vi "RTS Read Point File.vi"(8 "Error In":errorcluster, 11 "Path":path) -> (0 "Error Out":errorcluster, 2 "Array 2":string[](array[string]), 3 "Point File":T1[](array[typedef]))   [LabVIEW 2018]
uses:
  Type Definitions/RTS Point File.ctl
  <vilib>/Utility/file.llb/Read Delimited Spreadsheet (string).vi
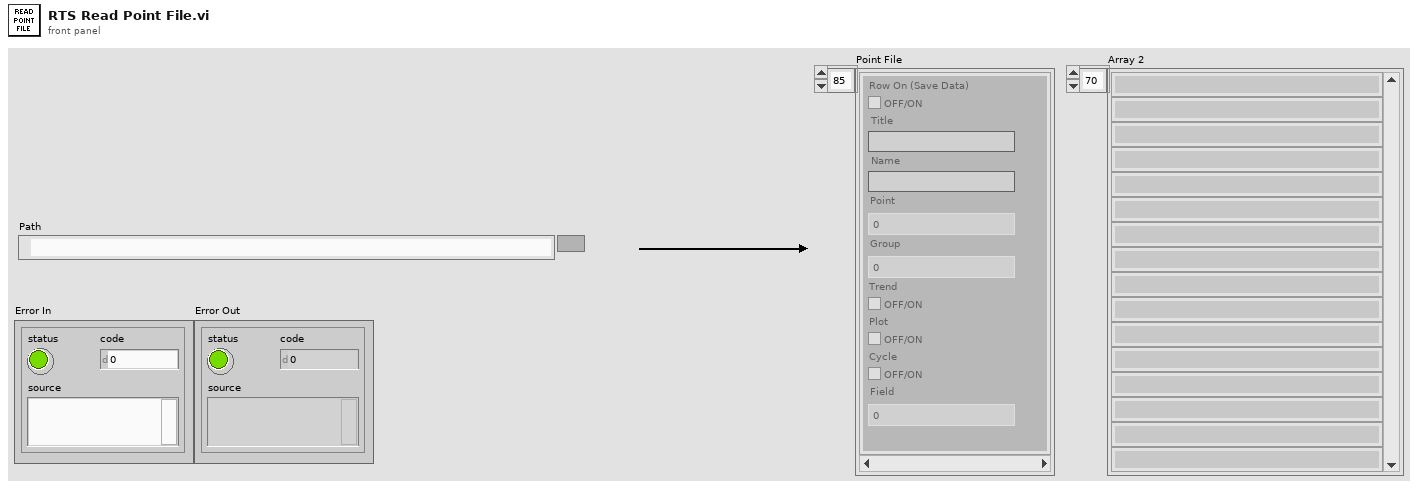
[diagram p1: front panel]
types:
  T1 = typedef "RTS Point File.ctl" = cluster{"Title":string, "Name":string, "Point":u8, "Plot":bool, "Trend":bool, "Cycle":bool, "Field":u8, "Row On (Save Data)":bool, "Group":u8}
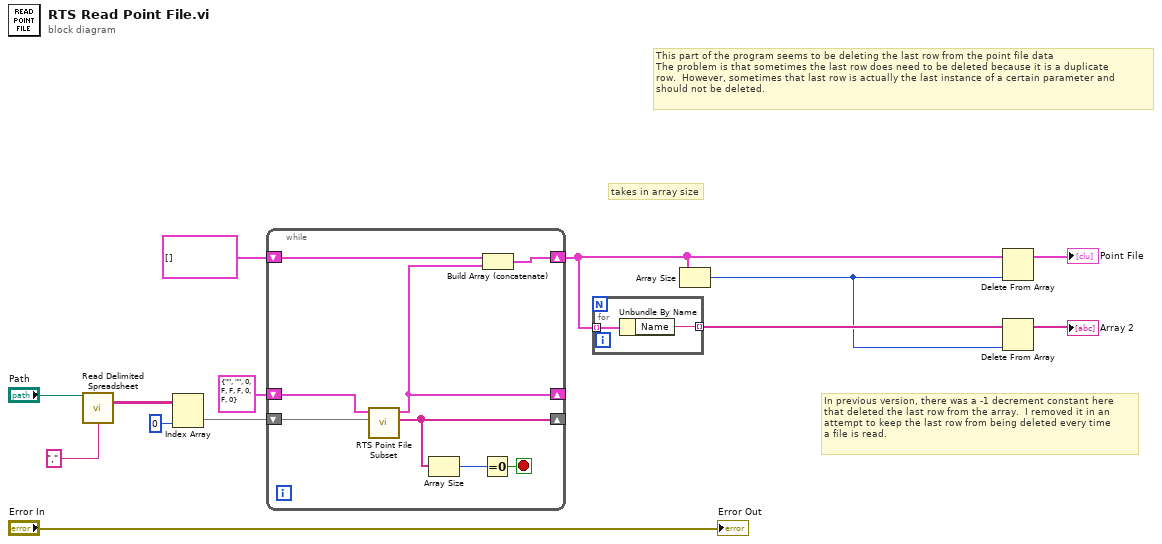
[diagram p0: block diagram]
diagram:
  # "In previous version, there was a -1 decrement constant here\nthat deleted the last row from the array.  I removed it in an\nattempt to keep the last row from being deleted every time \na file is read."
  # "takes in array size"
  # "This part of the program seems to be deleting the last row from the point file data\nThe problem is that sometimes the last row does need to be deleted because it is a duplicate\nrow.  However, sometimes that last row is actually the last instance of a certain parameter and \nshould not be deleted."
  n1 = call-poly <vilib>:"Read Delimited Spreadsheet.vi"("file path (dialog if empty)"="Path", "delimiter (\\t)"="," ("delimiter (\\t)")) -> ("all rows"=w12:string[][])  [unwired: 8 in, 5 out]
  n2 = Index Array(array=w12, index (col)=0 ("disabled index (col)")) -> (element=w6:string[])  [unwired: 1 in]
  n3 = while {
    shift-right: [w19] -> _
    shift-left: w6 -> [w21]
    shift-right: [w16] -> _
    shift-left: T1 {"Title"="", "Name"="", "Point"=0, "Plot"=FALSE, "Trend"=FALSE, "Cycle"=FALSE, "Field"=0, "Row On (Save Data)"=FALSE, "Group"=0} ("Point File Input") -> [w20]
    shift-right: [w17] -> w5
    shift-left: T1[] [] -> [w18]
    stop <- w15 stop-if-true
    n4 = call "RTS Point File Subset.vi"("Data Input"=w21, "Point File Input"=w20) -> ("Next Subset"=w19:string[], "Point File Output"=w16:T1)  [unwired: 7 in, 1 out]
    n5 = Array Size(array=w19) -> (size(s)=w14:i32)
    n6 = Equal To 0?(x=w14) -> (x = 0?=w15:bool)
    n7 = Build Array (concatenate)(w18, w16) -> (w17:T1[])
  }
  n8 = for {
    tunnel: w5 -> [w23] mode=indexing
    tunnel: [w22] -> w3 mode=indexing
    n9 = Unbundle By Name(w23) -> ("Name"=w22:string)
  }
  n10 = Array Size(array=w5) -> (size(s)=w1:i32)
  n11 = Delete From Array(array=w5, index=w1) -> (array with subset deleted=→"Point File":T1[])  [unwired: 1 in, 1 out]
  n12 = Delete From Array(array=w3, index=w1) -> (array with subset deleted=→"Array 2":string[])  [unwired: 1 in, 1 out]
  "Error Out" <- "Error In"
